vi "Write.vi"(8 "error in (no error)":errorcluster, 9 "Data":u8[](array[numeric]) format="%x", 10 "ID":u32 format="%x", 11 "PCANUSB in":refnum<class "PCANUSB.lvclass">) -> (0 "error out":errorcluster, 3 "PCANUSB out":refnum<class "PCANUSB.lvclass">)   [LabVIEW 2024, in "PCANUSB.lvclass"]
uses:
  PCANUSB.lvclass
  PCANUSB.lvclass/PCANUSB.ctl
  PCAN/CAN Communication.llb/CAN MSG Cluster.ctl
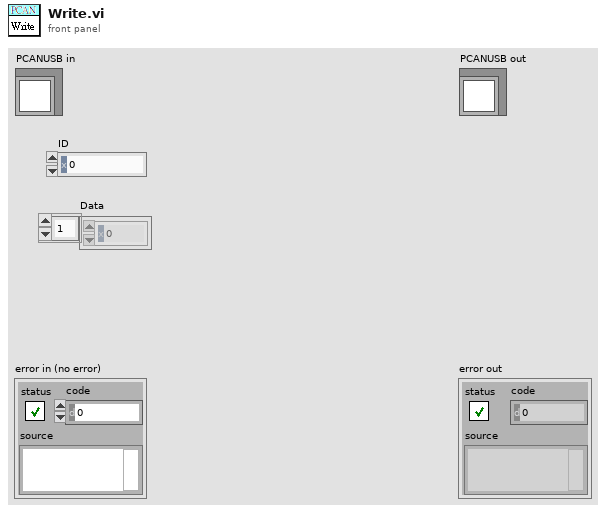
[diagram p1: front panel]
types:
  T1 = typedef "CAN MSG Cluster.ctl" = cluster{"ID":u32, "MSG type":u8, "DLC":u8, "DATA":u8[]}
  T2 = typedef "TPCANHandle.ctl" = enum16{"PCAN_NONEBUS  0x000", "PCAN_ISABUS1  0x21", "PCAN_ISABUS2  0x22", "PCAN_ISABUS3  0x23", "PCAN_ISABUS4  0x24", "PCAN_ISABUS5  0x25", "PCAN_ISABUS6  0x26", "PCAN_ISABUS7  0x27", "PCAN_ISABUS8  0x28", "PCAN_DNGBUS1  0x31", "PCAN_PCIBUS1  0x41", "PCAN_PCIBUS1  0x42", "PCAN_PCIBUS1  0x43", "PCAN_PCIBUS1  0x44", "PCAN_PCIBUS1  0x45", "PCAN_PCIBUS1  0x46", "PCAN_PCIBUS1  0x47", "PCAN_PCIBUS1  0x48", "PCAN_PCIBUS1  0x409", "PCAN_PCIBUS1  0x40A", "PCAN_PCIBUS1  0x40B", "PCAN_PCIBUS1  0x40C", "PCAN_PCIBUS1  0x40D", "PCAN_PCIBUS1  0x40E", "PCAN_PCIBUS1  0x40F", "PCAN_PCIBUS1  0x410", "PCAN_USBBUS1  0x51", "PCAN_USBBUS2  0x52", "PCAN_USBBUS3  0x53", "PCAN_USBBUS4  0x54", "PCAN_USBBUS5  0x55", "PCAN_USBBUS6  0x56", "PCAN_USBBUS7  0x57", "PCAN_USBBUS8  0x58", "PCAN_USBBUS9  0x509", "PCAN_USBBUS10  0x50A", "PCAN_USBBUS11  0x50B", "PCAN_USBBUS12  0x50C", "PCAN_USBBUS13  0x50D", "PCAN_USBBUS14  0x50E", "PCAN_USBBUS15  0x50F", "PCAN_USBBUS16  0x510", "PCAN_PCCBUS1  0x61", "PCAN_PCCBUS2  0x62", "PCAN_LANBUS1  0x801", "PCAN_LANBUS2  0x802", "PCAN_LANBUS3  0x803", "PCAN_LANBUS4  0x804", "PCAN_LANBUS5  0x805", "PCAN_LANBUS6  0x806", "PCAN_LANBUS7  0x807", "PCAN_LANBUS8  0x808", "PCAN_LANBUS9  0x809", "PCAN_LANBUS10  0x80A", "PCAN_LANBUS11  0x80B", "PCAN_LANBUS12  0x80C", "PCAN_LANBUS13  0x80D", "PCAN_LANBUS14  0x80E", "PCAN_LANBUS15  0x80F", "PCAN_LANBUS16  0x810"}
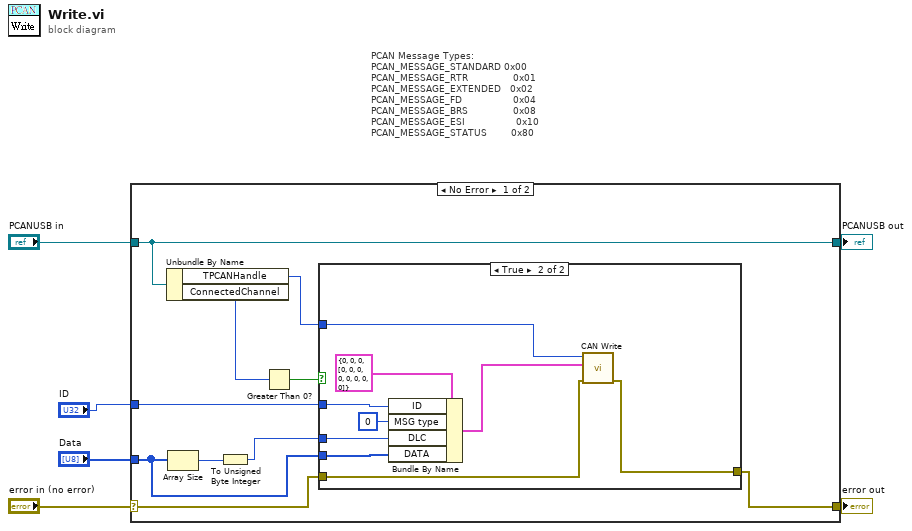
[diagram p0: block diagram]
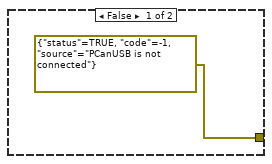
[diagram p2: hidden frame]
diagram:
  # "PCAN Message Types:\nPCAN_MESSAGE_STANDARD 0x00\nPCAN_MESSAGE_RTR               0x01\nPCAN_MESSAGE_EXTENDED   0x02\nPCAN_MESSAGE_FD                 0x04\nPCAN_MESSAGE_BRS               0x08\nPCAN_MESSAGE_ESI                 0x10\nPCAN_MESSAGE_STATUS        0x80"
  n1 = case shown="No Error" "error in (no error)" {
    selector: "error in (no error)" -> [w15 w28]
    tunnel: [w14 w28] -> w5
    tunnel: [w13 w27] -> w3
    tunnel: "PCANUSB in" -> [w13 w27]
    tunnel: "ID" -> [w11 _]
    tunnel: "Data" -> [w8 _]
    frame No Error {
      n2 = Unbundle By Name(w13) -> ("TPCANHandle"=w7:T2, "ConnectedChannel"=w12:u8)
      n3 = Array Size(array=w8) -> (size(s)=w10:i32)
      n4 = To Unsigned Byte Integer(number=w10) -> (unsigned 8bit integer=w9:u8)
      n5 = Greater Than 0?(x=w12) -> (x > 0?=w16:bool)
      n6 = case shown="True" w16 {
        tunnel: w15 -> [_ w25]
        tunnel: [errorcluster {"status"=TRUE, "code"=-1, "source"="PCanUSB is not connected"} ("error constant") w26] -> w14
        tunnel: w11 -> [_ w22]
        tunnel: w9 -> [_ w20]
        tunnel: w8 -> [_ w19]
        tunnel: w7 -> [_ w18]
        frame False {
        }
        frame True {
          n7 = Bundle By Name(cluster=T1 {"ID"=0, "MSG type"=0, "DLC"=0, "DATA"=[0, 0, 0, 0, 0, 0, 0, 0]} ("CAN_Message"), "ID"=w22, "MSG type"=u8 0, "DLC"=w20, "DATA"=w19) -> (w23:T1)
          n8 = call "CAN Write.vi"("error in (no error)"=w25, "CAN_Message"=w23, "TPCANHandle"=w18) -> ("error out"=w26:errorcluster)  [unwired: 7 in, 1 out]
        }
      }
    }
    frame Error {
    }
  }
  "error out" <- w5
  "PCANUSB out" <- w3
